vi "CameraStreamAttribute.vi"() -> ()   [LabVIEW 2020]
uses:
  <vilib>/userDefined/High Color/IMAQdx.ctl
  <vilib>/vision/driver/NI_Vision_Acquisition_Software.lvlib
  <resource>/objmgr/imaqdx.rc
panel:
  out "ValueString":string
  in  "Bit Depth (0)":u32
  out "EnumStrings[]":string[](array[string])
  in  "Session In":T1
  out "Image":T2(plugin-control)
  in  "Stop":bool
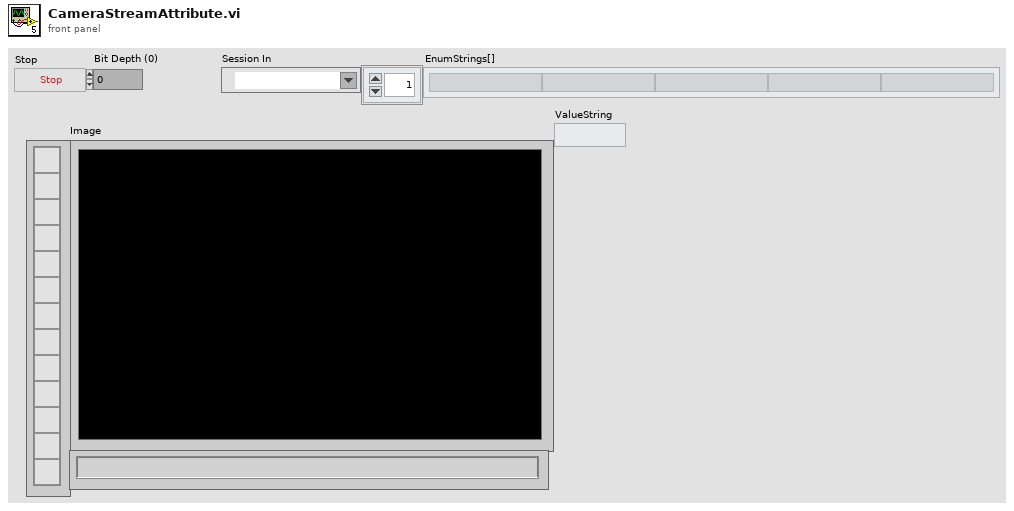
[diagram p1: front panel]
types:
  T1 = typedef "IMAQdx.ctl" = refnum<k21>
  T2 = typedef "IMAQ Image.ctl" = refnum<image>
  T3 = typedef "Image Type" = u32
  T4 = typedef "Color (U64)" = cluster{"Plane 3 (Blue)":u16, "Plane 2 (Green)":u16, "Plane 1 (Red)":u16, "Plane 4 (alpha)":u16}
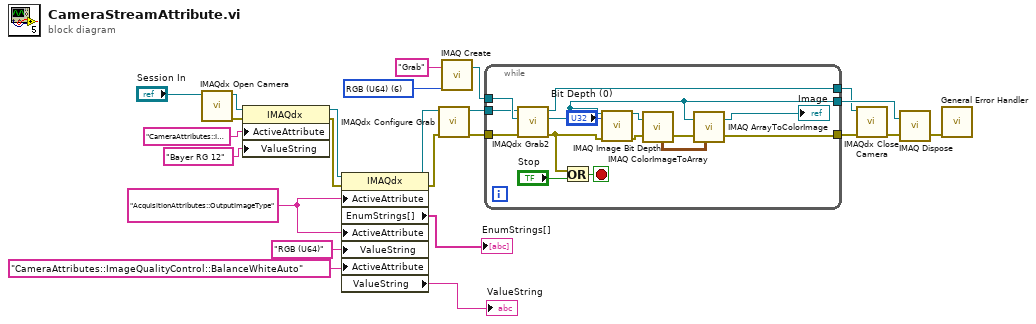
[diagram p0: block diagram]
diagram:
  w7 = "AcquisitionAttributes::OutputImageType" ("ActiveAttribute")
  w9 = T3 6 items=["Grayscale (U8)", "Grayscale (I16)", "Grayscale (SGL)", "Complex (CSG)", "RGB (U32)", "HSL (U32)", "RGB (U64)", "Grayscale (U16)"] ("Image Type")
  n1 = call <vilib>:"IMAQdx Open Camera.vi"("Session In"="Session In") -> ("error out"=w12:errorcluster, "Session Out"=w13:T1)  [unwired: 9 in]
  n2 = property class="IMAQdx"(reference=w13, error in=w12, "ActiveAttribute"="CameraAttributes::ImageFormatControl::PixelFormat", "ValueString"="Bayer RG 12") -> (reference out=w11:T1, error out=w4:errorcluster)
  n3 = property class="IMAQdx"(reference=w11, error in=w4, "ActiveAttribute"=w7, "ActiveAttribute"=w7, "ValueString"="RGB (U64)", "ActiveAttribute"="CameraAttributes::ImageQualityControl::BalanceWhiteAuto") -> (reference out=w5:T1, error out=w3:errorcluster, "EnumStrings[]"=→"EnumStrings[]":string[], "ValueString"=→"ValueString":string)
  n4 = call <vilib>:"IMAQdx Configure Grab.vi"("error in"=w3, "Session In"=w5) -> ("error out"=w15:errorcluster, "Session Out"=w16:T1)  [unwired: 8 in]
  n5 = call "IMAQ Create"("Image Name"="Grab", "Image Type"=w9) -> ("New Image"=w23:T2)  [unwired: 3 in, 1 out]
  n6 = while {
    tunnel: w15 -> [w34]
    tunnel: w23 -> [w37]
    tunnel: w16 -> [w36]
    tunnel: [w25] -> w21
    tunnel: [w26] -> w22
    tunnel: [w35] -> w20
    stop <- w38 stop-if-true
    n7 = call <vilib>:"IMAQdx Grab2.vi"("error in"=w34, "Image In"=w37, "Session In"=w36) -> ("error out"=w29:errorcluster, "Image Out"=w26:T2, "Session Out"=w35:T1)  [unwired: 5 in, 1 out]
    n8 = Or(x=w29, y="Stop") -> (x .or. y?=w38:bool)
    n9 = call "IMAQ Image Bit Depth"("Image"=w26, "Bit Depth (0)"="Bit Depth (0)", "error in (no error)"=w29) -> ("Image Out"=w33:T2, "error out"=w28:errorcluster)  [unwired: 10 in, 1 out]
    n10 = call "IMAQ ColorImageToArray"("Image"=w33, "error in (no error)"=w28) -> ("error out"=w30:errorcluster, "Image Pixels (U64)"=w31:T4[][])  [unwired: 2 in, 1 out]
    n11 = call "IMAQ ArrayToColorImage"("Image"=w26, "Image Pixels (U64)"=w31, "error in (no error)"=w30) -> ("Image Out"=→"Image":T2, "error out"=w25:errorcluster)  [unwired: 2 in]
  }
  n12 = call <vilib>:"IMAQdx Close Camera.vi"("error in"=w21, "Session In"=w20) -> ("error out"=w19:errorcluster)  [unwired: 9 in]
  n13 = call "IMAQ Dispose"("Image"=w22, "error in (no error)"=w19) -> ("error out"=w18:errorcluster)  [unwired: 4 in]
  n14 = call <vilib>:"General Error Handler.vi"("error in (no error)"=w18) -> ()  [unwired: 10 in, 5 out]
